vi "URI to VI name.vi"(11 "URI":string) -> (3 "VI name":string)   [LabVIEW 2019, in "HTTP Server.lvlib"]
uses:
  HTTP Server.lvlib
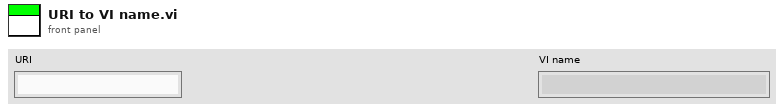
[diagram p1: front panel]
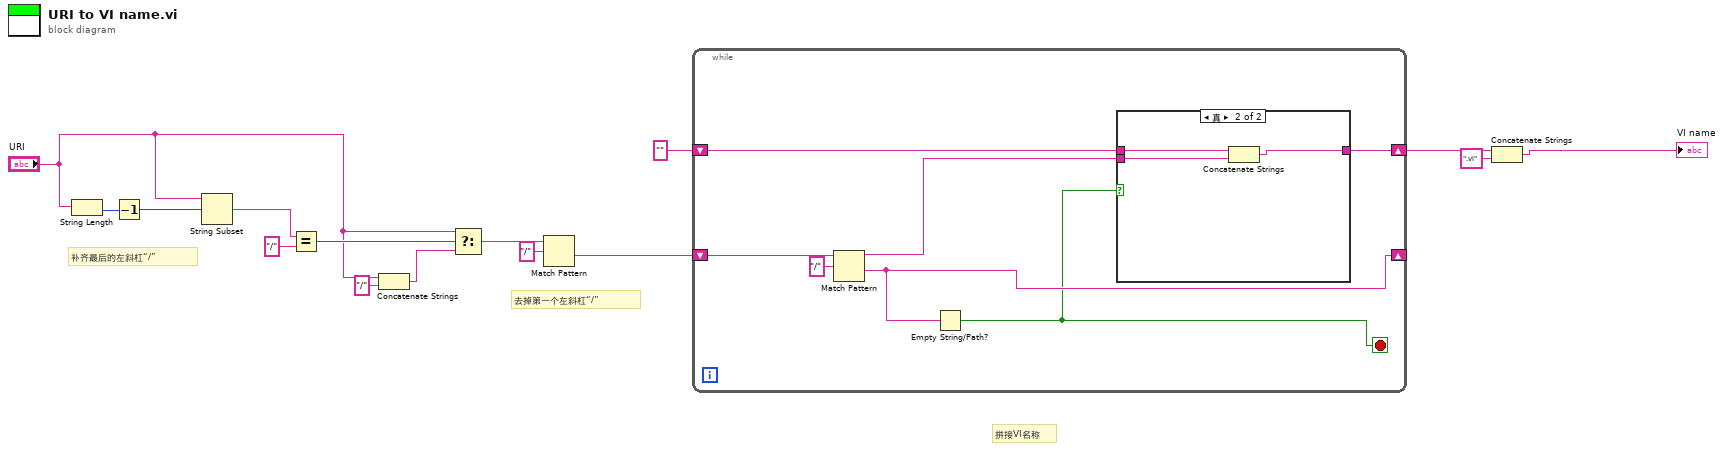
[diagram p0: block diagram]
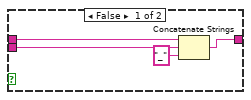
[diagram p2: hidden frame]
diagram:
  # "拼接VI名称"
  # "去掉第一个左斜杠“/”"
  # "补齐最后的左斜杠“/”"
  n1 = String Length(string="URI") -> (length=w15:i32)
  n2 = Decrement(x=w15) -> (x-1=w14:i32)
  n3 = String Subset(string="URI", offset (0)=w14) -> (substring=w13:string)  [unwired: 1 in]
  n4 = Equal?(x=w13, y="/") -> (x = y?=w11:bool)
  n5 = Concatenate Strings("URI", "/" ("字符串")) -> (w9:string)
  n6 = Select(t="URI", s=w11, f=w9) -> (s? t:f=w8:string)
  n7 = Match Pattern(string=w8, regular expression="/" ("正则表达式")) -> (after substring=w5:string)  [unwired: 1 in, 3 out]
  n8 = while {
    shift-right: [w17] -> _
    shift-left: w5 -> [w20]
    shift-right: [w21] -> w4
    shift-left: "" -> [w22]
    stop <- w16 stop-if-true
    n9 = Match Pattern(string=w20, regular expression="/" ("正则表达式")) -> (before substring=w18:string, after substring=w17:string)  [unwired: 1 in, 2 out]
    n10 = Empty String/Path?(string/path=w17) -> (empty?=w16:bool)
    n11 = case shown="真" w16 {
      tunnel: w22 -> [w26 w29]
      tunnel: [w25 w27] -> w21
      tunnel: w18 -> [w24 w28]
      frame False {
        n12 = Concatenate Strings(w26, w24, "_" ("字符串")) -> (w25:string)
      }
      frame True {
        n13 = Concatenate Strings(w29, w28) -> (w27:string)
      }
    }
  }
  n14 = Concatenate Strings(w4, ".vi" ("字符串")) -> (→"VI name":string)
